vi "CDMA_cpich.vi"(8 "error in (no error)":errorcluster caption="错误输入（无错误）", 11 "Path":path) -> (0 "error out":errorcluster caption="错误输出", 1 "data_q":cdb[](array[numeric]), 2 "data_i":cdb[](array[numeric]), 3 "Path Out":path)   [LabVIEW 2015]
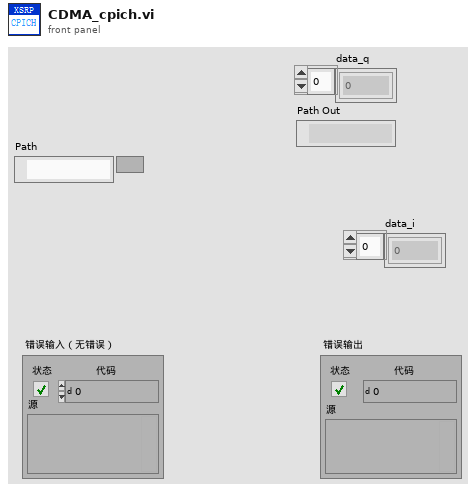
[diagram p1: front panel]
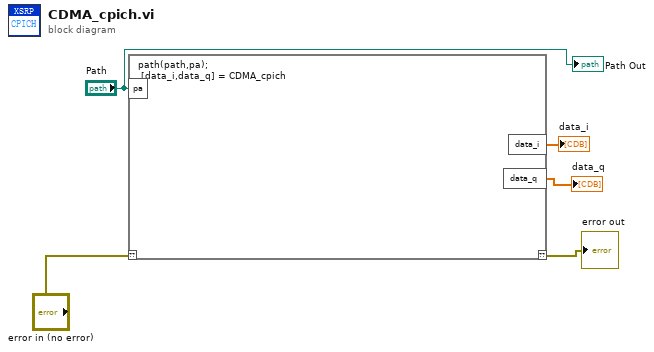
[diagram p0: block diagram]
diagram:
  n1 = script code="path(path,pa);\n [data_i,data_q] = CDMA_cpich"("??"="error in (no error)", "pa"="Path") -> ("??"=→"error out":errorcluster, "data_i"=→"data_i":cdb[], "data_q"=→"data_q":dbl[])
  "Path Out" <- "Path"
